vi "SVT Running Leq Sound Level (1 Ch).vi"(6 "restart averaging (F)":bool, 8 "error in (no error)":errorcluster, 9 "integration time [s]":dbl=1.0 format="%.2f", 11 "scaled signal [EU]":waveform(dbl)={"t0"=timestamp(0 s since 1904-01-01), "dt"=1.0, "Y"=[0.0]}) -> (0 "error out":errorcluster, 1 "actual integration time [s]":dbl=nan format="%.2f", 2 "unit label":string, 3 "running Leq sound level [dB EU]":dbl=nan format="%.2f")   [LabVIEW 2017]
doc: "Computes the running equivalent continuous sound level (Leq) of <B>scaled signal [EU]</B>. A new running Leq value is returned each time you call this VI. You can use this polymorphic VI to compute the running Leq for a single channel or for N channels. The data type you wire to the <B>scaled signal [EU]</B> input determines the polymorphic instance to use."
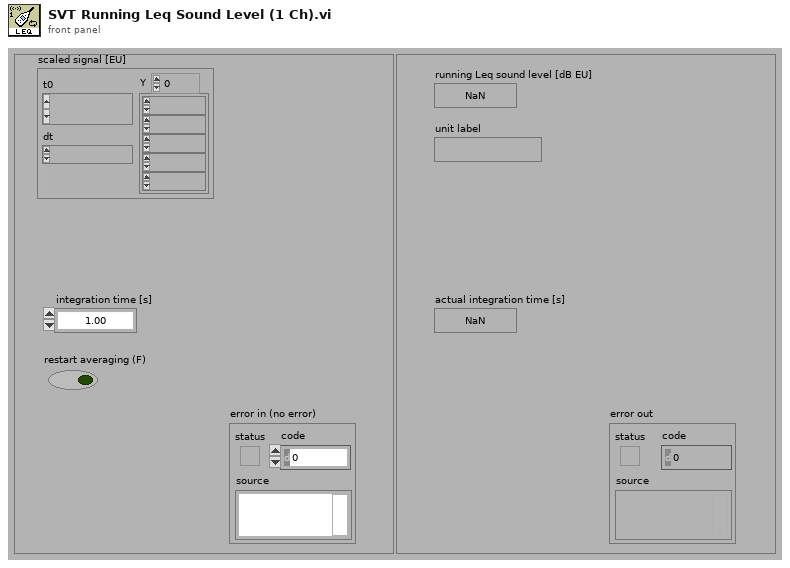
[diagram p1: front panel]
types:
  T1 = enum16{"RMS", "Running RMS", "Exp avg  ", "Dec exp avg ", "Peak", "Crest"}
  T2 = enum16{"Reset filter", "Restart averaging", "Continue processing"}
  T3 = typedef "svc_Channel Info.ctl" = cluster{"sensor sensitivity":dbl, "engineering units":T4, "dB reference":dbl, "custom label":string, "weighting filter":T5, "pregain":dbl}
  T4 = typedef "svc_Engineering Units Text Ring.ctl" = u16
  T5 = typedef "svc_Weighting Filter Text Ring.ctl" = u16
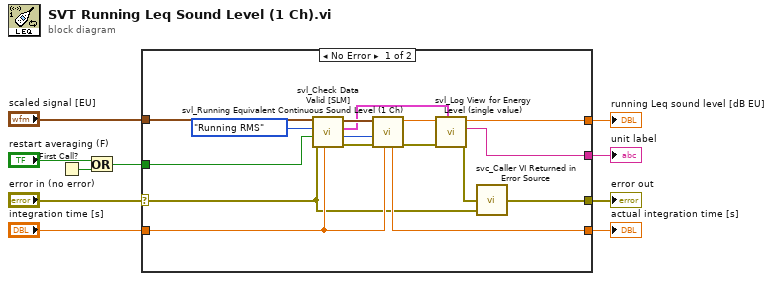
[diagram p0: block diagram]
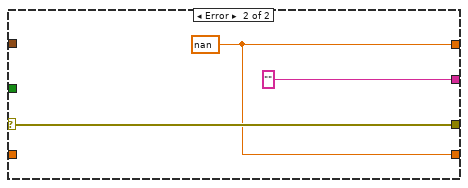
[diagram p2: hidden frame]
diagram:
  n1 = First Call?() -> (First Call?: T/F=w6:bool)
  n2 = Or(x="restart averaging (F)", y=w6) -> (x .or. y?=w2:bool)
  n3 = case shown="No Error" "error in (no error)" {
    selector: "error in (no error)" -> [w11 w29]
    tunnel: [w21 w29] -> w10
    tunnel: [w25 "" ("unit label")] -> w9
    tunnel: [w22 w27] -> w8
    tunnel: "integration time [s]" -> [w16 _]
    tunnel: [w18 w27] -> w4
    tunnel: "scaled signal [EU]" -> [w14 _]
    tunnel: w2 -> [w19 _]
    frame No Error {
      n4 = call <vilib>:"svl_Check Data Valid [SLM].vi"("integration time [s]"=w16, "error in (no error)"=w11, "restart averaging (F)"=w19, "Level Analysis"=T1."Running RMS", "scaled signal [EU]"=w14) -> ("error out"=w20:errorcluster, "processing state"=w17:T2, "channel info"=w12:T3, "dup scaled signal [EU]"=w13:waveform(dbl))  [unwired: 3 in]
      n5 = call <vilib>:"svl_Running Equivalent Continuous Sound Level (1 Ch).vi"("integration time [s]"=w16, "error in (no error)"=w20, "processing state"=w17, "scaled signal"=w13) -> ("error out"=w24:errorcluster, "Running Leq"=w23:dbl, "actual integration time [s]"=w18:dbl)  [unwired: 5 in]
      n6 = call <vilib>:"svl_Log View for Energy Level (single value).vi"("channel info"=w12, "error in (no error)"=w24, "energy level [EU^2 rms]"=w23) -> ("error out"=w26:errorcluster, "unit label"=w25:string, "energy level [EU^2 rms]"=w22:dbl)  [unwired: 6 in]
      n7 = call <vilib>:"svc_Caller VI Returned in Error Source.vi"("warning input to caller"=w11, "error in (no error)"=w26) -> ("error out"=w21:errorcluster)  [unwired: 3 in]
    }
    frame Error {
      w27 = nan ("energy level [EU^2 rms]")
    }
  }
  "running Leq sound level [dB EU]" <- w8
  "unit label" <- w9
  "error out" <- w10
  "actual integration time [s]" <- w4
